vi "FFT UI.vi"() -> ()   [LabVIEW 2020]
doc: "This VI provides a UI for the \"LabVIEW FPGA FFT.vi\" example."
uses:
  <vilib>/FPGAPlugInAG/cRIO-9054/niLvFpga_Open_cRIO-9054.vi
  <vilib>/rvi/interface/common/dynamic/niFpgaDynamicAddResources.vi
  <vilib>/rvi/Analysis/host/Private/Sample Rate To Loop Time (ticks).vi
  <vilib>/Utility/error.llb/Error Cluster From Error Code.vi
  <vilib>/rvi/errors/niLvFpgaAdjustHostInterfaceError.vi
  <vilib>/FPGAPlugInAG/Dynamic/niLvFpga_Close_Dynamic.vi
  <vilib>/rvi/interface/nirviOpenFPGA/nirviOpenFPGA.xnode
  FPGA Bitfiles/fft_FPGATarget2_LabVIEWFPGAFFT_Ii2GKIkw6TE.lvbitx
  LabVIEW FPGA FFT.vi
  <vilib>/rvi/interface/nirviReadWriteControl/nirviReadWriteControl.xnode
  <vilib>/rvi/interface/nirviMethod/nirviMethod.xnode
  <vilib>/rvi/interface/nirviCloseFPGA/nirviCloseFPGA.xnode
  <vilib>/rvi/Analysis/host/Public/NI_FpgaMspHost.lvlib
  <vilib>/FPGAPlugInAG/Dynamic/niLvFpga_ReadFifo_Dynamic.vi
  <vilib>/rvi/errors/niLvFpgaMergeErrorWithErrorCode.vi
  NiFpgaLv.dll
  <vilib>/rvi/interface/Simulation/niFpgaSimulationCallBeginRW.vi
panel:
  out "Signal":waveform(dbl)(graph)={"t0"=timestamp(0 s since 1904-01-01), "dt"=2e-05, "Y"=[]}
  out "FFT Spectrum":waveform(dbl)(graph)={"t0"=timestamp(0 s since 1904-01-01), "dt"=195.3125, "Y"=[]}
  in  "Stop":bool
  in  "Frequency (Hz)":dbl=4000.0 min=0.0 format="%#_7p"
  in  "Sample rate (S/s)":dbl=50000.0 min=1.0 format="%#_7p"
  out "Invalid Sample Rate":bool
  # "Overview: Demonstrates the use of the LabVIEW FPGA FFT function for custom in-hardware signal processing\nRequirements: LabVIEW FPGA Module, NI-RIO\nInstructions: Run the VI"
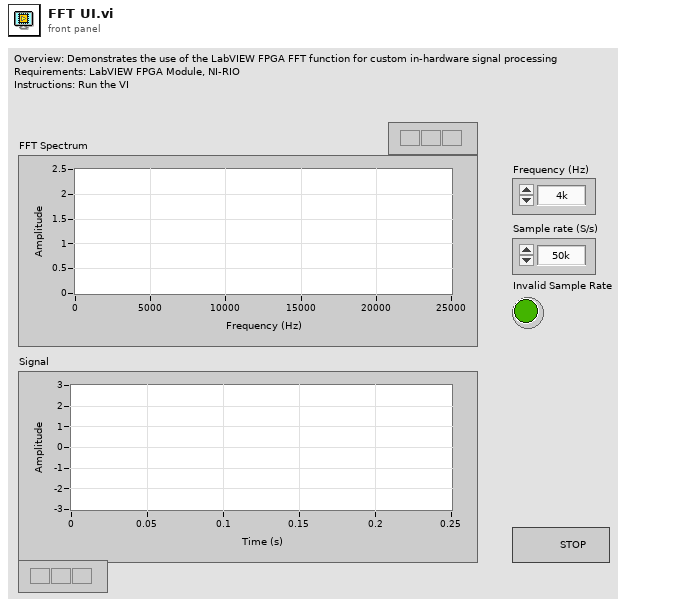
[diagram p1: front panel]
types:
  T1 = typedef "niFpgaViExecutionMode.ctl" = enum16{"FPGA Target", "Simulation (Simulated I/O)", "Simulation (Real I/O)", "Third-Party Simulation"}
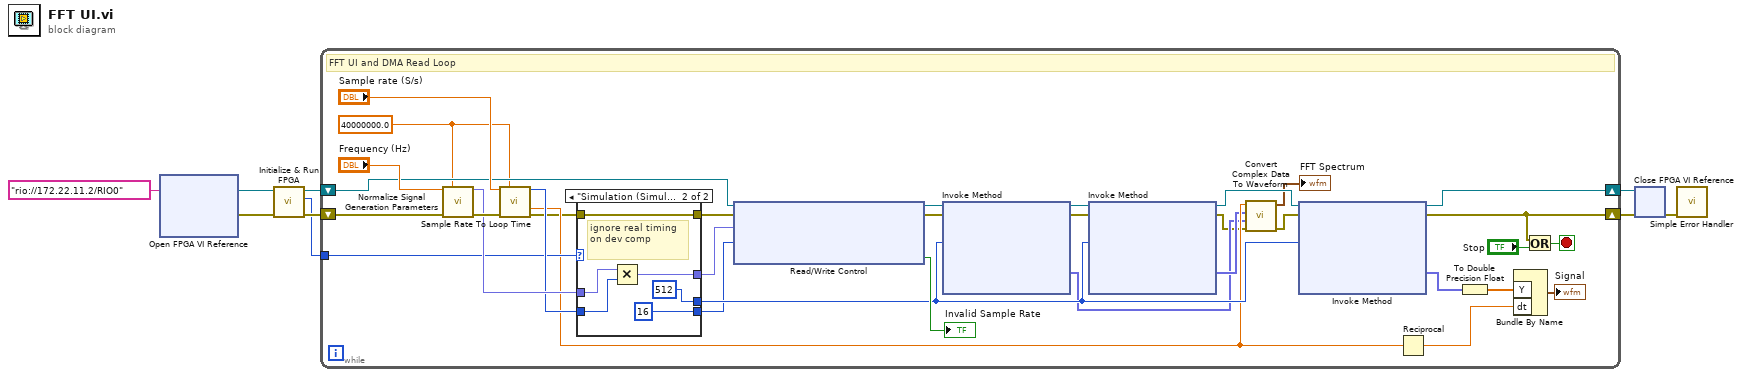
[diagram p0: block diagram]
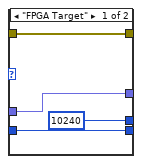
[diagram p2: hidden frame]
diagram:
  n1 = xnode "Open FPGA VI Reference"("resource name"=tag "rio://172.22.11.2/RIO0") -> ("FPGA VI Reference Out"=w4:refnum<k20>, "error out"=w3:errorcluster)  [unwired: 1 in]
  n2 = call "Initialize & Run FPGA.vi"("error in (no error)"=w3, "Refnum in"=w4) -> ("error out"=w6:errorcluster, "FPGA VI Execution Mode"=w5:T1, "Refnum out"=w7:refnum<k20>)  [unwired: 7 in]
  n3 = while {
    shift-right: [w40] -> w9
    shift-left: w7 -> [w22]
    shift-right: [w24] -> w8
    shift-left: w6 -> [w23]
    tunnel: w5 -> [w19]
    stop <- w34 stop-if-true
    w21 = 40000000.0 ("FPGA clock rate (Hz)")
    # "FFT UI and DMA Read Loop"
    n4 = call <vilib>:"Normalize Signal Generation Parameters.vi"("frequency (Hz)"="Frequency (Hz)", "FPGA clock rate (Hz)"=w21, "error in (no error)"=w23) -> ("frequency (periods/tick)"=w38:fxp<+,32,0>, "error out"=w39:errorcluster)  [unwired: 7 in, 4 out]
    n5 = call-poly <vilib>:"Sample Rate To Loop Time.vi"("sample rate (S/s)"="Sample rate (S/s)", "FPGA clock rate (Hz)"=w21, "error in (no error)"=w39) -> ("count (ticks/S)"=w33:u32, "actual sample rate (S/s)"=w18:dbl, "error out"=w13:errorcluster)  [unwired: 10 in]
    n6 = case shown="\"Simulation (Simulated I/O)\", Default" w19 {
      tunnel: [u32 10240 ("Number of Elements") u32 512 ("Number of Elements")] -> w27
      tunnel: w38 -> [w46 w52]
      tunnel: [w46 w51] -> w29
      tunnel: w33 -> [w45 w50]
      tunnel: [w45 u32 16 ("count (ticks/S)")] -> w20
      tunnel: w13 -> [w44 w48]
      tunnel: [w44 w48] -> w12
      frame "FPGA Target" {
      }
      frame "Simulation (Simulated I/O)", Default {
        # "ignore real timing on dev comp"
        n7 = Multiply(x=w52, y=w50) -> (x*y=w51:fxp<+,32,0>)
      }
    }
    n8 = xnode "Read/Write Control"("FPGA VI Reference In"=w22, "error in"=w12, "Frequency (periods/tick)"=w29, "Requested Sample Period (ticks)"=w20) -> ("FPGA VI Reference Out"=w32:refnum<k20>, "error out"=w25:errorcluster, "Invalid Period"=→"Invalid Sample Rate":bool)
    n9 = xnode "Invoke Method"("FPGA VI Reference In"=w32, "error in"=w25, "Number of Elements"=w27) -> ("FPGA VI Reference Out"=w42:refnum<k20>, "error out"=w26:errorcluster, "Data"=w16:fxp<+/-,25,14>[])  [unwired: 1 in, 1 out]
    n10 = xnode "Invoke Method"("FPGA VI Reference In"=w42, "error in"=w26, "Number of Elements"=w27) -> ("FPGA VI Reference Out"=w41:refnum<k20>, "error out"=w15:errorcluster, "Data"=w17:fxp<+/-,25,14>[])  [unwired: 1 in, 1 out]
    n11 = call "Convert Complex Data To Waveform.vi"("error in"=w15, "Real Data"=w16, "Imaginary Data"=w17, "Sample Rate (S/s)"=w18) -> ("error out"=w14:errorcluster, "Waveform"=→"FFT Spectrum":waveform(dbl))  [unwired: 6 in]
    n12 = xnode "Invoke Method"("FPGA VI Reference In"=w41, "error in"=w14, "Number of Elements"=w27) -> ("FPGA VI Reference Out"=w40:refnum<k20>, "error out"=w24:errorcluster, "Data"=w43:fxp<+/-,16,5>[])  [unwired: 1 in, 1 out]
    n13 = Reciprocal(x=w18) -> (1/x=w36:dbl)
    n14 = To Double Precision Float(number=w43) -> (double precision float=w37:dbl[])
    n15 = Bundle By Name("Y"=w37, "dt"=w36) -> (→"Signal":waveform(dbl))  [unwired: 1 in]
    n16 = Or(x=w24, y="Stop") -> (x .or. y?=w34:bool)
  }
  n17 = xnode "Close FPGA VI Reference"("FPGA VI Reference In"=w9, "error in"=w8) -> ("error out"=w2:errorcluster)
  n18 = call <vilib>:"Simple Error Handler.vi"("error in (no error)"=w2) -> ()  [unwired: 4 in, 5 out]
